vi "6_3.vi"() -> ()   [LabVIEW 2020]
panel:
  in  "Numerisch 4":dbl
  in  "Numerisch 3":dbl
  in  "Numerisch 2":dbl
  in  "Numerisch":dbl
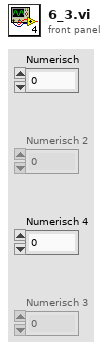
[diagram p1: front panel]
types:
  T1 = enum8{"Enabled", "Disabled", "Disabled and Grayed Out"}[]
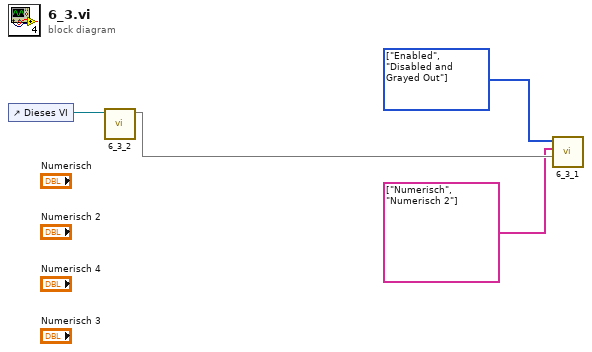
[diagram p0: block diagram]
diagram:
  w1 = T1 [enum."Enabled", enum."Disabled and Grayed Out"] items=["Enabled", "Disabled", "Disabled and Grayed Out"] ("Deaktiviert")
  n1 = control-ref of="Dieses VI"() -> (w4:refnum<vi>)
  n2 = call "6_3_2.vi"("VI (Eingang)"=w4) -> ("Map"=w3:map{string, refnum<vi>})  [unwired: 10 in]
  n3 = call "6_3_1.vi"("Map"=w3, "Schlüssel"=string[] ["Numerisch", "Numerisch 2"], "Deaktiviert"=w1) -> ()  [unwired: 9 in]
